vi "populate sonde row cluster from sonde data cluster.vi"(2 "Time Value":dbl, 7 "Initialize \nInitial Value \nCluster":bool, 8 "error in (no error)":errorcluster, 9 "Sonde Parameters \nInitial Values":T3 {"Salinity Initial" format="%_2f"; "Temp Initial" format="%_2f"; "ORP  Initial" format="%_2f"; "pH Initial" format="%_2f"; "DO Initial" format="%_2f"; "SC Initial" format="%_2f"}, 10 "Sample Sheet Data Row Cluster":T1={"Head"=0.0, "Depth"=0.0, "comment string"="", "Sonde Data Cluster"={"Cumulative\nVolume"=100.0, "Specific\nConductance"=2.0, "Dissolved\nOxygen"=3.0, "pH"=4.0, "ORP"=5.0, "Temp"=26.0, "Salinity"=7.0}} {"Sonde Data Cluster"."Salinity" format="%_3g"; "Sonde Data Cluster"."Temp" format="%_2g"; "Sonde Data Cluster"."ORP" format="%_4g"; "Sonde Data Cluster"."pH" format="%_4g"; "Sonde Data Cluster"."Dissolved\nOxygen" format="%_4g"; "Sonde Data Cluster"."Specific\nConductance" format="%_4g"; "Sonde Data Cluster"."Cumulative\nVolume" format="%#_4g"}, 11 "Sonde Parameters \nTolerance Limits":T6 {"Salinity %" format="%_2f%%"; "Temp %" format="%_2f%%"; "ORP %" format="%_2f%%"; "pH %" format="%_2f%%"; "DO %" format="%_2f%%"; "SC %" format="%_2f%%"}) -> (0 "error out":errorcluster, 1 "Cluster":T4 {"Salinity"."%" format="%_2f%%"; "Salinity"."Value" format="%_4g"; "Temperature"."%" format="%_2f%%"; "Temperature"."Value" format="%_4g"; "ORP"."%" format="%_2f%%"; "ORP"."Value" format="%_4g"; "pH"."%" format="%_2f%%"; "pH"."Value" format="%_4g"; "Dissolved Oxygen"."%" format="%_2f%%"; "Dissolved Oxygen"."Value" format="%_4g"; "Sp. Conductance"."%" format="%_2f%%"; "Sp. Conductance"."Value" format="%_4g"; "Cumulative\nVolume" format="%#_4g"}, 6 "Sonde Parameters \nInitial Values Out":T3 {"Salinity Initial" format="%_2f"; "Temp Initial" format="%_2f"; "ORP  Initial" format="%_2f"; "pH Initial" format="%_2f"; "DO Initial" format="%_2f"; "SC Initial" format="%_2f"})   [LabVIEW 2016]
uses:
  activeXtest/activeXtest 2015 Folder/sonde cluster from excel.ctl
  Sonde Value Percent Tol.ctl
  activeXtest/activeXtest 2015 Folder/sample data row cluster.ctl
  activeXtest/activeXtest 2015 Folder/sonde cluster.ctl
panel:
  in  "Final":bool
  in  "Input Cluster for % calculation":T4 caption="Cluster" {"Salinity"."%" format="%_2f%%"; "Salinity"."Value" format="%_4g"; "Temperature"."%" format="%_2f%%"; "Temperature"."Value" format="%_4g"; "ORP"."%" format="%_2f%%"; "ORP"."Value" format="%_4g"; "pH"."%" format="%_2f%%"; "pH"."Value" format="%_4g"; "Dissolved Oxygen"."%" format="%_2f%%"; "Dissolved Oxygen"."Value" format="%_4g"; "Sp. Conductance"."%" format="%_2f%%"; "Sp. Conductance"."Value" format="%_4g"; "Cumulative\nVolume" format="%#_4g"}
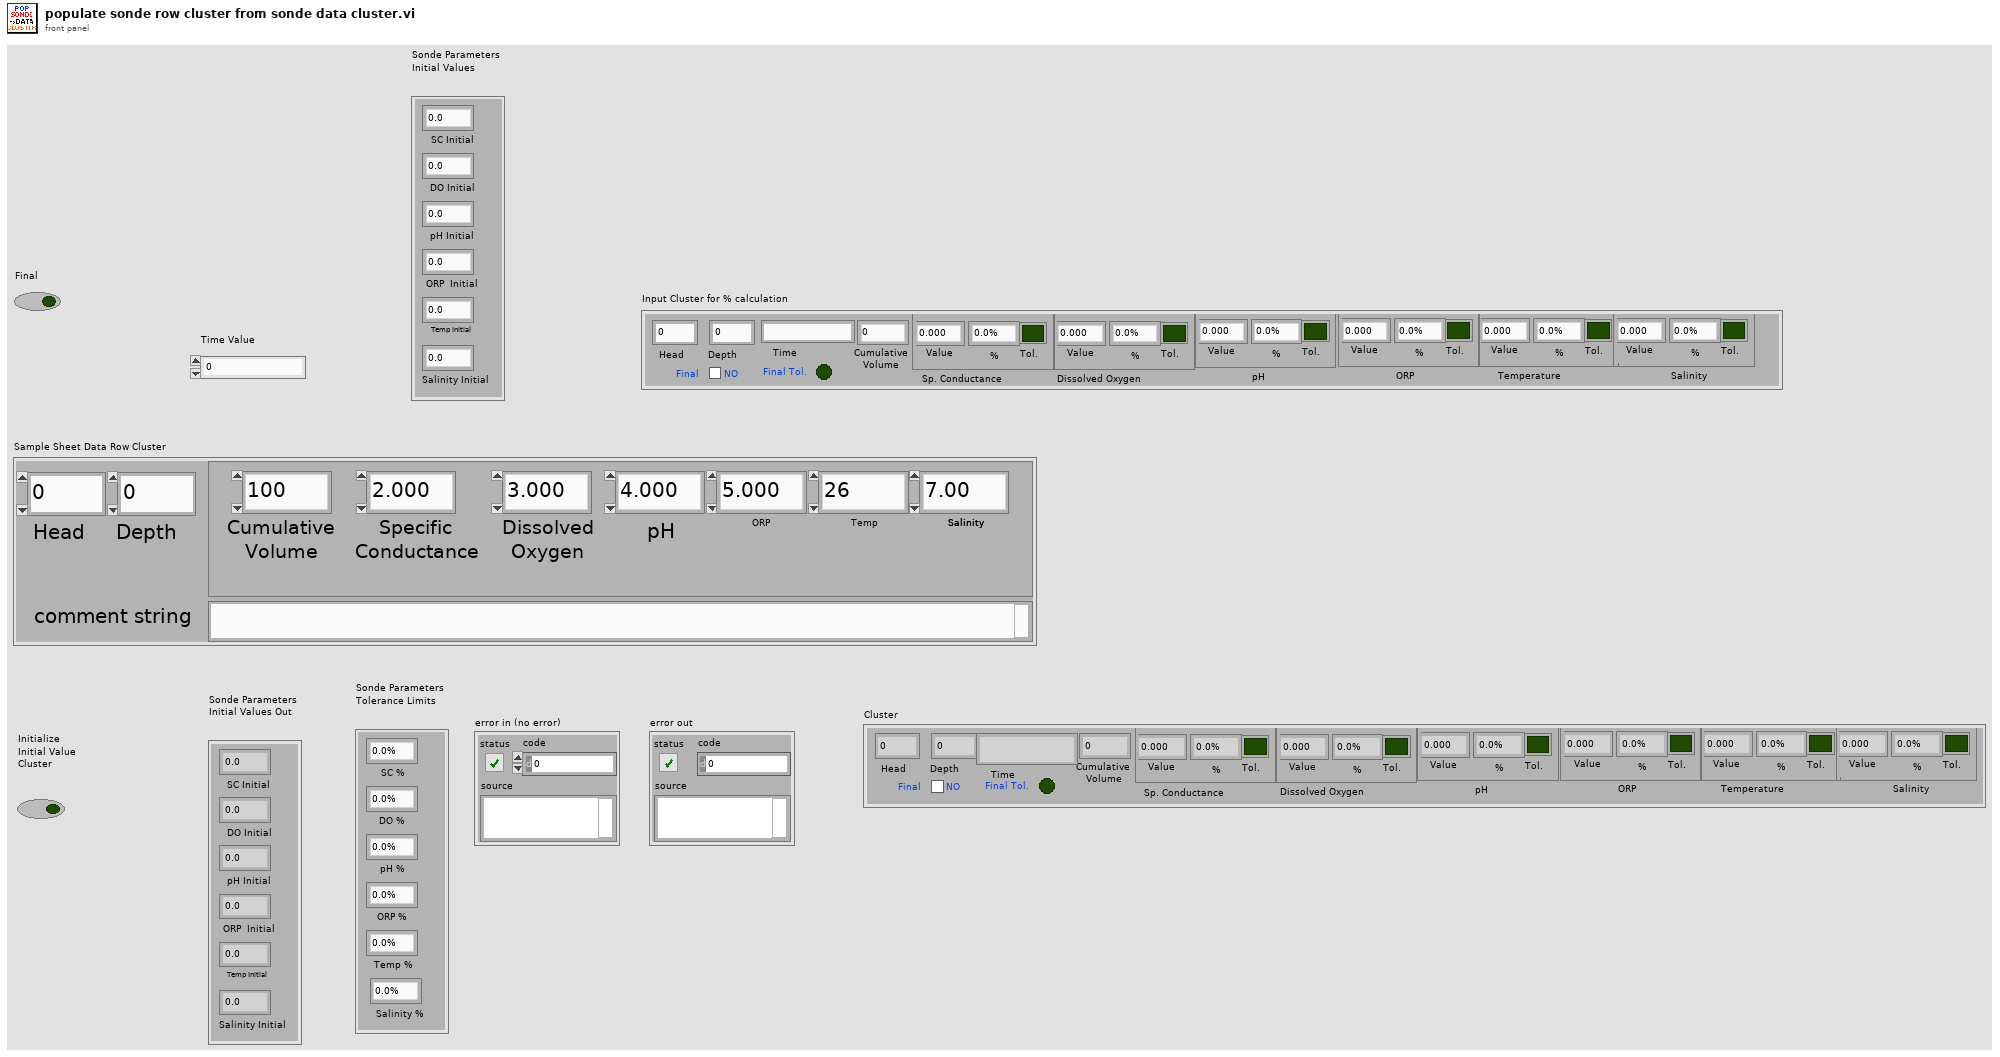
[diagram p1: front panel]
types:
  T1 = typedef "sample data row cluster.ctl" = cluster{"Head":dbl, "Depth":dbl, "comment string":string, "Sonde Data Cluster":T2}
  T2 = typedef "sonde cluster.ctl" = cluster{"Cumulative\nVolume":dbl, "Specific\nConductance":dbl, "Dissolved\nOxygen":dbl, "pH":dbl, "ORP":dbl, "Temp":dbl, "Salinity":dbl}
  T3 = cluster{"SC Initial ":dbl, "DO Initial ":dbl, "pH Initial  ":dbl, "ORP  Initial":dbl, "Temp Initial":dbl, "Salinity Initial ":dbl}
  T4 = typedef "sonde cluster from excel.ctl" = cluster{"Head":dbl, "Depth":dbl, "Time":string, "Cumulative\nVolume":dbl, "Sp. Conductance":T5, "Dissolved Oxygen":T5, "pH":T5, "ORP":T5, "Temperature":T5, "Salinity":T5, "Final Tol.":bool, "Final":bool}
  T5 = typedef "Sonde Value Percent Tol.ctl" = cluster{"Value":dbl, "%":dbl, "Tol.":bool}
  T6 = cluster{"SC %":dbl, "DO %":dbl, "pH % ":dbl, "ORP % ":dbl, "Temp % ":dbl, "Salinity %":dbl}
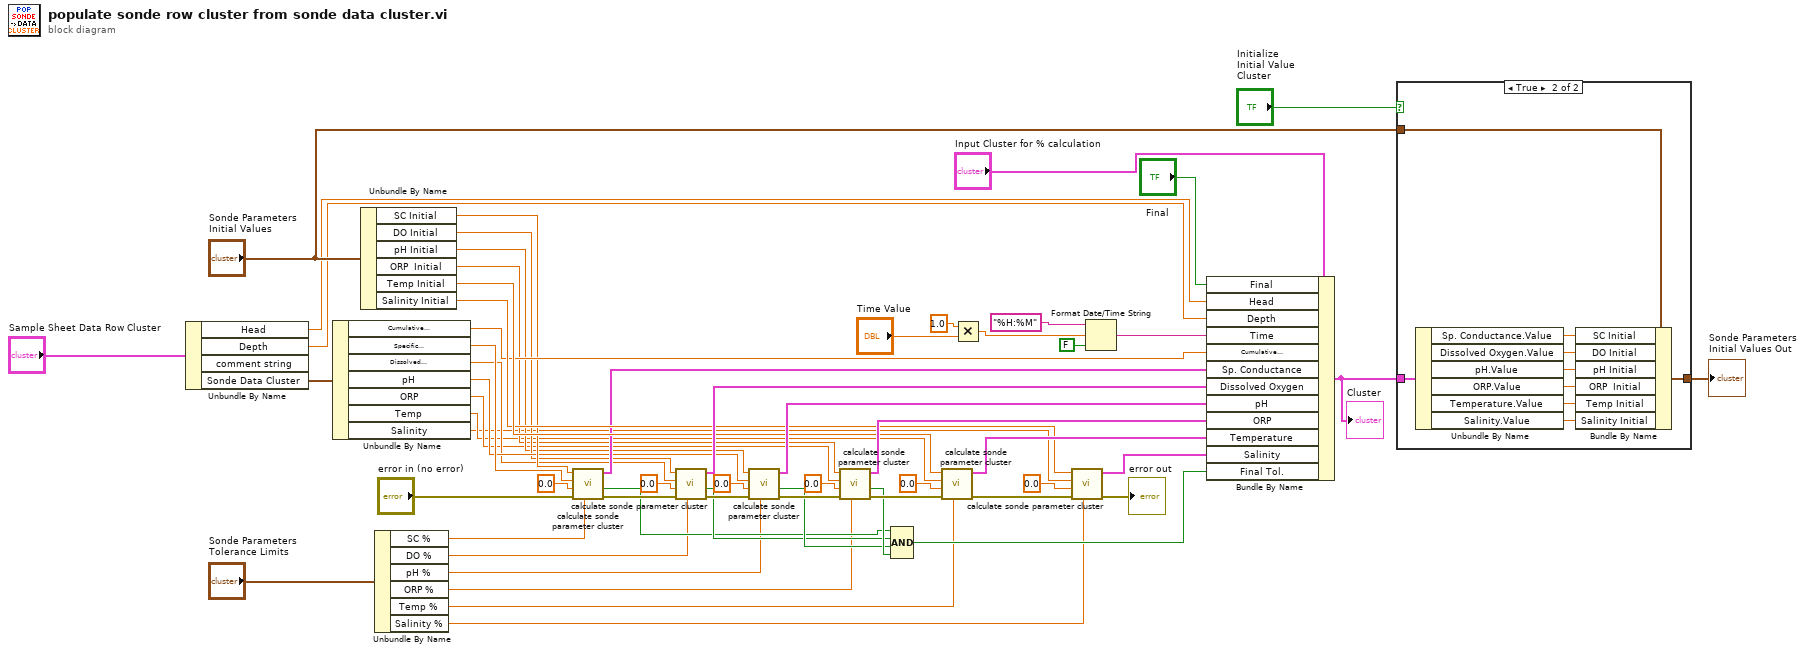
[diagram p0: block diagram]
diagram:
  n1 = Unbundle By Name("Sample Sheet Data Row Cluster") -> ("Head"=w29:dbl, "Depth"=w28:dbl, "Sonde Data Cluster"=w27:T2)  [unwired: 1 out]
  n2 = Unbundle By Name(w27) -> ("Cumulative\nVolume"=w26:dbl, "Specific\nConductance"=w21:dbl, "Dissolved\nOxygen"=w15:dbl, "pH"=w17:dbl, "ORP"=w8:dbl, "Temp"=w5:dbl, "Salinity"=w3:dbl)
  n3 = Unbundle By Name("Sonde Parameters \nInitial Values") -> ("SC Initial"=w24:dbl, "DO Initial"=w13:dbl, "pH Initial"=w11:dbl, "ORP  Initial"=w9:dbl, "Temp Initial"=w35:dbl, "Salinity Initial"=w34:dbl)
  n4 = Unbundle By Name("Sonde Parameters \nTolerance Limits") -> ("SC %"=w23:dbl, "DO %"=w12:dbl, "pH %"=w16:dbl, "ORP %"=w7:dbl, "Temp %"=w41:dbl, "Salinity %"=w40:dbl)
  n5 = call "calculate sonde parameter cluster.vi"("tolerance limit"=w23, "error in (no error)"="error in (no error)", "Read % value"=0.0, "Read Value"=w21, "Initial Value"=w24) -> ("error out"=w20:errorcluster, "Tolerance"=w19:bool, "Cluster Out"=w22:T5)  [unwired: 3 in, 1 out]
  n6 = call "calculate sonde parameter cluster.vi"("tolerance limit"=w12, "error in (no error)"=w20, "Read % value"=0.0, "Read Value"=w15, "Initial Value"=w13) -> ("error out"=w58:errorcluster, "Tolerance"=w49:bool, "Cluster Out"=w44:T5)  [unwired: 3 in, 1 out]
  n7 = call "calculate sonde parameter cluster.vi"("tolerance limit"=w16, "error in (no error)"=w58, "Read % value"=0.0, "Read Value"=w17, "Initial Value"=w11) -> ("error out"=w57:errorcluster, "Tolerance"=w50:bool, "Cluster Out"=w45:T5)  [unwired: 3 in, 1 out]
  n8 = call "calculate sonde parameter cluster.vi"("tolerance limit"=w7, "error in (no error)"=w57, "Read % value"=0.0, "Read Value"=w8, "Initial Value"=w9) -> ("error out"=w56:errorcluster, "Tolerance"=w51:bool, "Cluster Out"=w46:T5)  [unwired: 3 in, 1 out]
  n9 = Compound Arithmetic op=AND(w19, w49, w50, w51) -> (w52:bool)
  n10 = call "calculate sonde parameter cluster.vi"("tolerance limit"=w41, "error in (no error)"=w56, "Read % value"=0.0, "Read Value"=w5, "Initial Value"=w35) -> ("error out"=w55:errorcluster, "Cluster Out"=w47:T5)  [unwired: 3 in, 2 out]
  n11 = Multiply(x=1.0, y="Time Value") -> (x*y=w39:dbl)
  n12 = call "calculate sonde parameter cluster.vi"("tolerance limit"=w40, "error in (no error)"=w55, "Read % value"=0.0, "Read Value"=w3, "Initial Value"=w34) -> ("error out"=→"error out":errorcluster, "Cluster Out"=w48:T5)  [unwired: 3 in, 2 out]
  n13 = Format Date/Time String(time format string (%c)="%H:%M", seconds (now)=w39, UTC format=FALSE) -> (date/time string=w43:string)
  n14 = Bundle By Name(cluster="Input Cluster for % calculation", "Final"="Final", "Head"=w29, "Depth"=w28, "Time"=w43, "Cumulative\nVolume"=w26, "Sp. Conductance"=w22, "Dissolved Oxygen"=w44, "pH"=w45, "ORP"=w46, "Temperature"=w47, "Salinity"=w48, "Final Tol."=w52) -> (w31:T4)
  "Cluster" <- w31
  n15 = case shown="True" "Initialize \nInitial Value \nCluster" {
    tunnel: "Sonde Parameters \nInitial Values" -> [w61 w70]
    tunnel: [w61 w69] -> w33
    tunnel: w31 -> [_ w68]
    frame False {
    }
    frame True {
      n16 = Unbundle By Name(w68) -> ("Sp. Conductance.Value"=w67:dbl, "Dissolved Oxygen.Value"=w66:dbl, "pH.Value"=w65:dbl, "ORP.Value"=w64:dbl, "Temperature.Value"=w63:dbl, "Salinity.Value"=w62:dbl)
      n17 = Bundle By Name(cluster=w70, "SC Initial"=w67, "DO Initial"=w66, "pH Initial"=w65, "ORP  Initial"=w64, "Temp Initial"=w63, "Salinity Initial"=w62) -> (w69:T3)
    }
  }
  "Sonde Parameters \nInitial Values Out" <- w33
